vi "WPI_EncoderGet.vi"(8 "error in (no error)":errorcluster, 11 "EncoderDevRef":T1={"DevStatus"={"status"=FALSE, "code"=0, "source"=""}, "EncoderIndex"=enum."Invalid", "CounterIndex"=enum."Ctr 1", "DistancePerCount"=2.0, "Decoding Type"=enum."4x"}) -> (0 "error out":errorcluster, 1 "Direction":bool, 2 "Distance":dbl, 3 "EncoderDevRef":T1={"DevStatus"={"status"=FALSE, "code"=0, "source"=""}, "EncoderIndex"=enum."Invalid", "CounterIndex"=enum."Ctr 1", "DistancePerCount"=2.0, "Decoding Type"=enum."4x"}, 4 "Rate":dbl, 6 "Stopped":bool)   [LabVIEW 2017]
doc: "Returns information about the count, direction, and period of the encoder you specify, as well as whether the encoder is stopped.\n\nThis software is licensed. Open the labview\\readme\\WPI Robotics Library Open Source License.txt file for more information."
uses:
  <vilib>/Rock Robotics/WPI/Encoder/WPI_EncoderDevRef.ctl
  <vilib>/Rock Robotics/SystemInterfaces/Encoder/FPGA_EncoderIdx.ctl
  <vilib>/Rock Robotics/SystemInterfaces/Counter/FPGA_CounterCtrSystemIndex.ctl
  <vilib>/Rock Robotics/WPI/Encoder/WPI_EncoderType.ctl
  <instrlib>/Maxon Encoder/HAIOL/Maxon Encoder.lvclass
  <vilib>/Rock Robotics/SystemInterfaces/Encoder/FPGA_EncoderOpen WO Configuration.vi
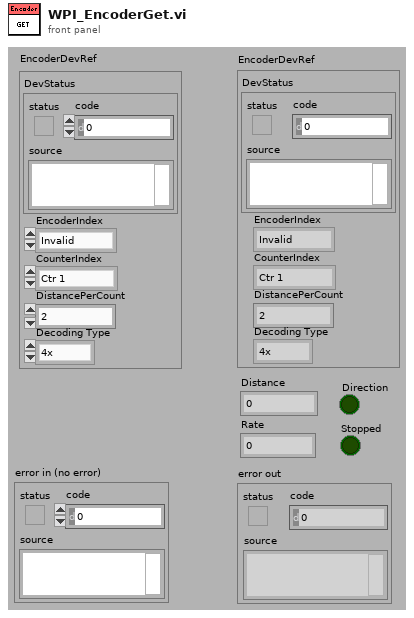
[diagram p1: front panel]
types:
  T1 = typedef "WPI_EncoderDevRef.ctl" = cluster{"DevStatus":errorcluster, "EncoderIndex":T2, "CounterIndex":T3, "DistancePerCount":dbl, "Decoding Type":T4}
  T2 = typedef "FPGA_EncoderIdx.ctl" = enum8{"Enc 0", "Enc 1", "Enc 2", "Enc 3", "Enc 4", "Enc 5", "Enc 6", "Enc 7", "Invalid"}
  T3 = typedef "FPGA_CounterCtrSystemIndex.ctl" = enum8{"Ctr 0", "Ctr 1", "Ctr 2", "Ctr 3", "Ctr 4", "Ctr 5", "Ctr 6", "Ctr 7", "Invalid"}
  T4 = typedef "WPI_EncoderType.ctl" = enum16{"1x", "2x", "4x"}
  T5 = typedef "FPGA_CounterCtrDevRef.ctl" = cluster{"DevStatus":errorcluster, "CntIndex":T3}
  T6 = typedef "FPGA_EncoderDevRef.ctl" = cluster{"EncoderIndex":T2, "DevStatus":errorcluster}
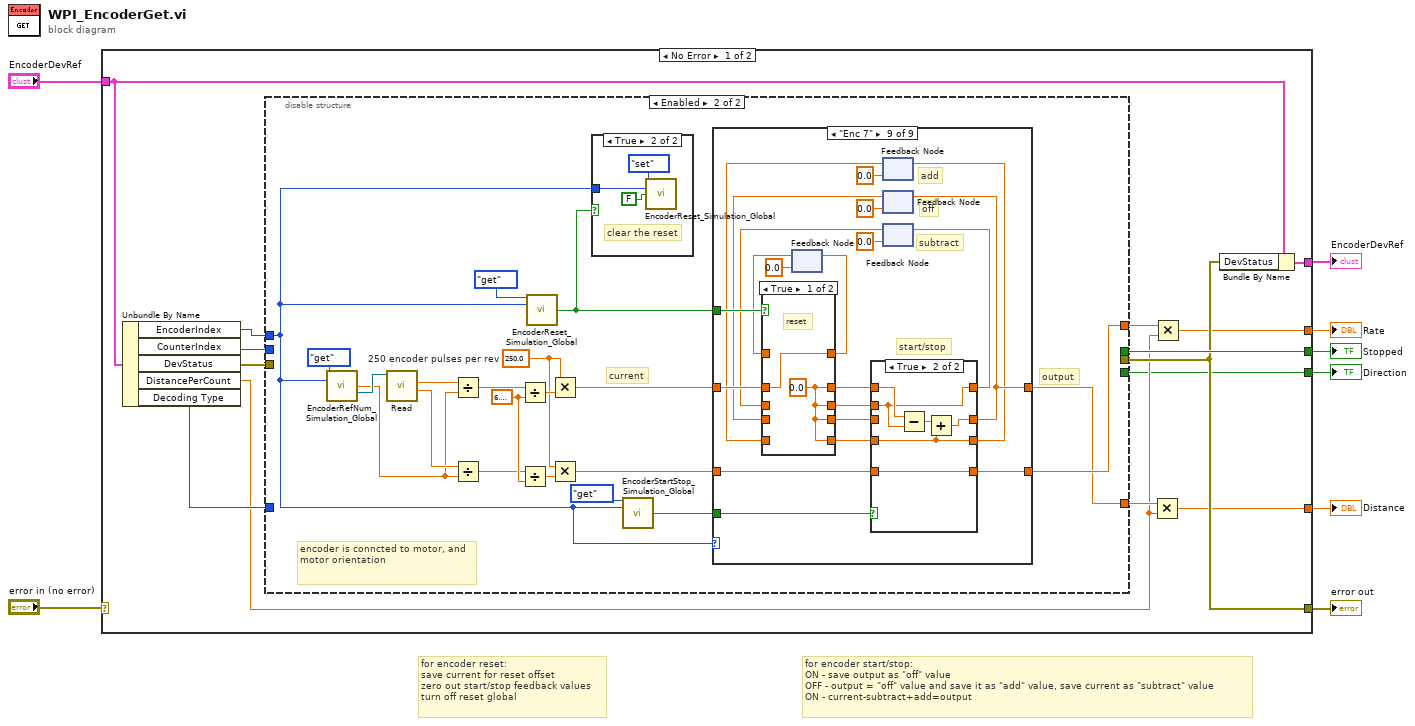
[diagram p0: block diagram]
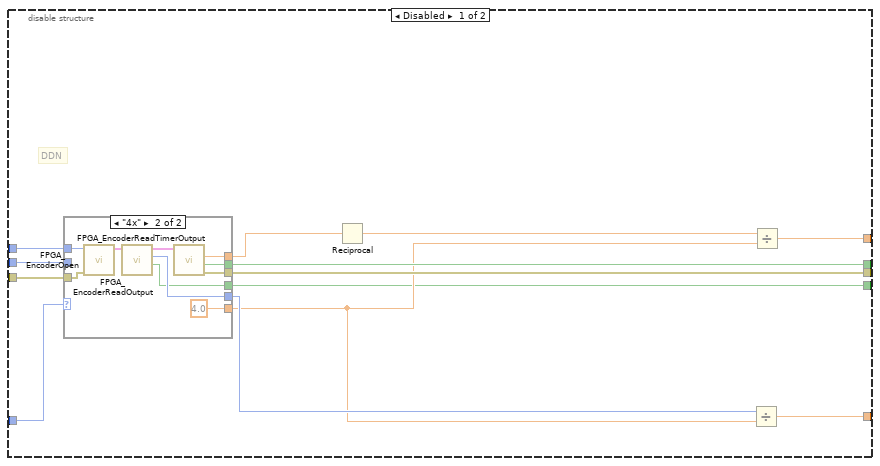
[diagram p2: hidden frame]
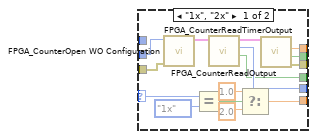
[diagram p3: hidden frame]
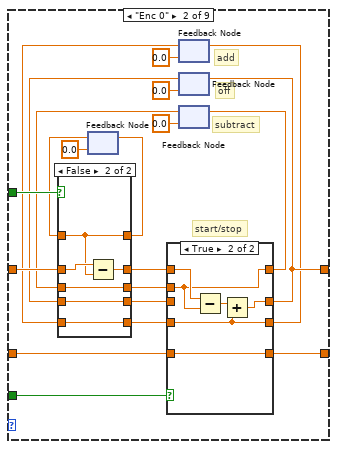
[diagram p6: hidden frame]
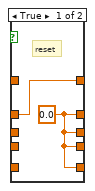
[diagram p7: hidden frame]
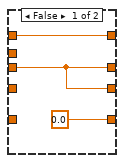
[diagram p8: hidden frame]
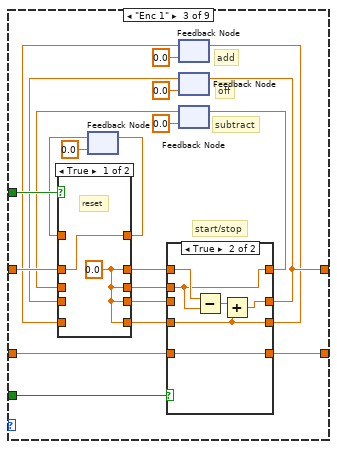
[diagram p9: hidden frame]
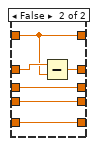
[diagram p10: hidden frame]
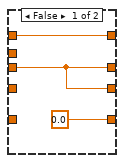
[diagram p11: hidden frame]
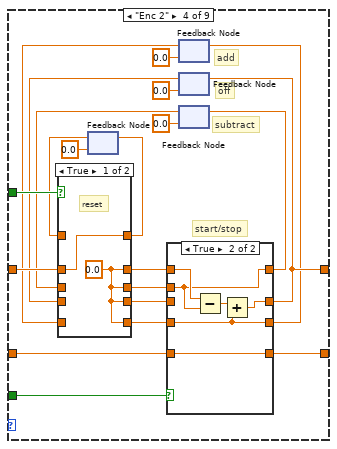
[diagram p12: hidden frame]
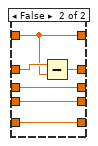
[diagram p13: hidden frame]
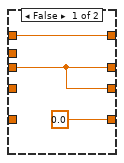
[diagram p14: hidden frame]
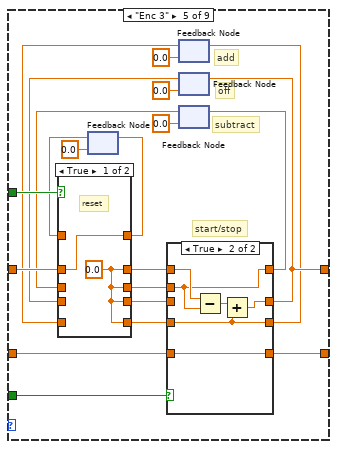
[diagram p15: hidden frame]
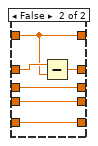
[diagram p16: hidden frame]
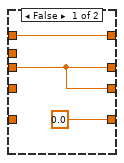
[diagram p17: hidden frame]
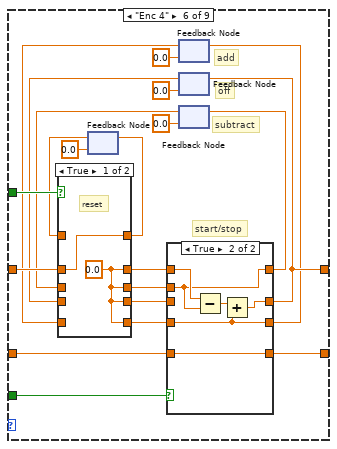
[diagram p18: hidden frame]
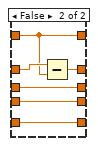
[diagram p19: hidden frame]
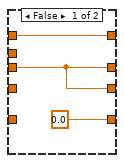
[diagram p20: hidden frame]
diagram:
  # "for encoder reset:\nsave current for reset offset\nzero out start/stop feedback values\nturn off reset global"
  # "for encoder start/stop:\nON - save output as \"off\" value\nOFF - output = \"off\" value and save it as \"add\" value, save current as \"subtract\" value\nON - current-subtract+add=output"
  n1 = case shown="No Error" "error in (no error)" {
    selector: "error in (no error)" -> [_ w390]
    tunnel: "EncoderDevRef" -> [w19 w392]
    tunnel: [w10 _] -> w4
    tunnel: [w15 w390] -> w6
    tunnel: [w22 w391] -> w5
    tunnel: [w12 _] -> w3
    tunnel: [w21 _] -> w2
    tunnel: [w11 _] -> w1
    frame No Error {
      n2 = Unbundle By Name(w19) -> ("EncoderIndex"=w9:T2, "CounterIndex"=w17:T3, "DevStatus"=w18:errorcluster, "DistancePerCount"=w13:dbl, "Decoding Type"=w16:T4)
      n3 = disable-structure shown="Enabled" {
        disable-tunnel: w9 -> [w35 w63]
        disable-tunnel: [w34 _] -> w21
        disable-tunnel: [w33 w62] -> w20
        disable-tunnel: w18 -> [w31 _]
        disable-tunnel: w17 -> [w30 _]
        disable-tunnel: w16 -> [w29 _]
        disable-tunnel: [w28 _] -> w15
        disable-tunnel: [w27 w65] -> w14
        disable-tunnel: [w23 _] -> w12
        frame Disabled {
          # "DDN"
          n4 = case shown="\"4x\"" w29 {
            selector: w29 -> [w49 _]
            tunnel: w35 -> [_ w60]
            tunnel: [w42 w58] -> w32
            tunnel: [w38 w56] -> w34
            tunnel: [w39 w55] -> w24
            tunnel: [w41 w54] -> w23
            tunnel: [w40 w53] -> w28
            tunnel: [w50 4.0] -> w25
            tunnel: w31 -> [w36 w51]
            tunnel: w30 -> [w37 _]
            frame "1x", "2x" {
              n5 = call <vilib>:"FPGA_CounterOpen WO Configuration.vi"("error in"=w36, "CntIndex"=w37) -> ("Ctr Ref"=w43:T5)  [unwired: 1 in, 8 out]
              n6 = Equal?(x=w49, y=WPI_EncoderType."1x") -> (x = y?=w45:bool)
              n7 = call <vilib>:"FPGA_CounterReadOutput.vi"("Ctr Ref in"=w43) -> ("Direction"=w41:bool, "Value"=w42:i32, "Ctr Ref out"=w44:T5)  [unwired: 1 in, 7 out]
              n8 = Select(t=1.0, s=w45, f=2.0) -> (s? t:f=w50:dbl)
              n9 = call <vilib>:"FPGA_CounterReadTimerOutput.vi"("Ctr Ref in"=w44) -> ("error out"=w40:errorcluster, "Stalled"=w38:bool, "Period (s)"=w39:dbl)  [unwired: 1 in, 7 out]
            }
            frame "4x" {
              n10 = call-poly <vilib>:"FPGA_EncoderOpen.vi"("DeviceStatus"=w51, "EncoderIndex"=w60) -> ("Encoder Reference"=w59:T6)  [unwired: 1 in, 8 out]
              n11 = call <vilib>:"FPGA_EncoderReadOutput.vi"("EncoderDevRef"=w59) -> ("Direction"=w54:bool, "Value"=w58:i32, "EncoderDevRef"=w57:T6)  [unwired: 1 in, 7 out]
              n12 = call <vilib>:"FPGA_EncoderReadTimerOutput.vi"("EncoderDevRef"=w57) -> ("error out"=w53:errorcluster, "Stalled"=w56:bool, "Period (s)"=w55:dbl)  [unwired: 1 in, 7 out]
            }
          }
          n13 = Reciprocal(x=w24) -> (1/x=w26:dbl)
          n14 = Divide(x=w32, y=w25) -> (x/y=w33:dbl)
          n15 = Divide(x=w26, y=w25) -> (x/y=w27:dbl)
        }
        frame Enabled {
          w75 = 250.0  # 250 encoder pulses per rev
          w76 = 6.283185307179586
          # "output"
          # "current"
          # "encoder is conncted to motor, and motor orientation"
          n16 = call <vilib>:"EncoderRefNum_Simulation_Global.vi"("menu"=enum16{"set", "get", "delete"}."get", "Encoder"=w63) -> ("Rate out"=w70:dbl, "Maxon Encoder Get"=w79:refnum<class "Maxon Encoder.lvclass">)  [unwired: 11 in, 1 out]
          n17 = call-dynamic "Read.vi"("Maxon Encoder in"=w79) -> ("Velocity (rad/Sec)"=w72:dbl, "Angular Position (rad)"=w74:dbl)  [unwired: 7 in, 2 out]
          n18 = Divide(x=w74, y=w70) -> (x/y=w73:dbl)
          n19 = Divide(x=w72, y=w70) -> (x/y=w71:dbl)
          n20 = Divide(x=w73, y=w76) -> (x/y=w78:dbl)
          n21 = Divide(x=w71, y=w76) -> (x/y=w77:dbl)
          n22 = call <vilib>:"EncoderReset_Simulation_Global.vi"("menu"=enum16{"set", "get", "delete"}."get", "Encoder Index"=w63) -> ("reset out"=w61:bool)  [unwired: 12 in, 1 out]
          n23 = Multiply(x=w75, y=w78) -> (x*y=w67:dbl)
          n24 = Multiply(x=w75, y=w77) -> (x*y=w66:dbl)
          n25 = case shown="True" w61 {
            tunnel: w63 -> [_ w83]
            frame False {
            }
            frame True {
              # "clear the reset"
              n26 = call <vilib>:"EncoderReset_Simulation_Global.vi"("menu"=enum16{"set", "get", "delete"}."set", "Encoder Index"=w83, "reset in"=FALSE) -> ()  [unwired: 11 in, 2 out]
            }
          }
          n27 = call <vilib>:"EncoderStartStop_Simulation_Global.vi"("menu"=enum16{"set", "get", "delete"}."get", "Encoder Index"=w63) -> ("start/stop out"=w68:bool)  [unwired: 12 in, 1 out]
          n28 = case shown="\"Enc 7\"" w63 {
            tunnel: w68 -> [_ w106 w144 w182 w220 w258 w296 w334 w372]
            tunnel: w67 -> [w85 w95 w133 w171 w209 w247 w285 w323 w361]
            tunnel: w66 -> [w84 w105 w143 w181 w219 w257 w295 w333 w371]
            tunnel: [w85 w99 w137 w175 w213 w251 w289 w327 w365] -> w62
            tunnel: [w84 w104 w142 w180 w218 w256 w294 w332 w370] -> w65
            tunnel: w61 -> [_ w97 w135 w173 w211 w249 w287 w325 w363]
            frame "Invalid" {
            }
            frame "Enc 0" {
              # "start/stop"
              # "add"
              # "subtract"
              # "off"
              n29 = feedback #1(0.0) -> (w93:dbl)
              n30 = feedback #2(0.0) -> (w91:dbl)
              n31 = feedback #3(0.0) -> (w89:dbl)
              n32 = feedback #4(0.0) -> (w86:dbl)
              n33 = case shown="False" w97 {
                tunnel: w95 -> [w108 w114]
                tunnel: [w107 w113] -> w94
                tunnel: w93 -> [_ w112]
                tunnel: [w108 w112] -> w92
                tunnel: w91 -> [_ w111]
                tunnel: [w107 w111] -> w90
                tunnel: [w107 w110] -> w88
                tunnel: w89 -> [_ w110]
                tunnel: [w107 w109] -> w87
                tunnel: w86 -> [_ w109]
                frame True {
                  w107 = 0.0
                  # "reset"
                }
                frame False {
                  n34 = Subtract(x=w114, y=w112) -> (x-y=w113:dbl)
                }
              }
              n35 = feedback-in #1(w92) -> ()
              n36 = case shown="True" w106 {
                tunnel: w94 -> [w116 w122]
                tunnel: [w115 w118] -> w99
                tunnel: w105 -> [_ w123]
                tunnel: [0.0 w123] -> w104
                tunnel: w88 -> [w115 _]
                tunnel: [w116 w121] -> w101
                tunnel: w87 -> [_ w121]
                tunnel: [w115 w119] -> w98
                tunnel: w90 -> [_ w119]
                frame False {
                }
                frame True {
                  n37 = Subtract(x=w122, y=w121) -> (x-y=w120:dbl)
                  n38 = Add(x=w120, y=w119) -> (x+y=w118:dbl)
                }
              }
              n39 = feedback-in #2(w98) -> ()
              n40 = feedback-in #3(w99) -> ()
              n41 = feedback-in #4(w101) -> ()
            }
            frame "Enc 1" {
              # "start/stop"
              # "add"
              # "subtract"
              # "off"
              n42 = feedback #5(0.0) -> (w131:dbl)
              n43 = feedback #6(0.0) -> (w129:dbl)
              n44 = feedback #7(0.0) -> (w127:dbl)
              n45 = feedback #8(0.0) -> (w124:dbl)
              n46 = case shown="True" w135 {
                tunnel: w133 -> [w146 w152]
                tunnel: [w145 w151] -> w132
                tunnel: w131 -> [_ w150]
                tunnel: [w146 w150] -> w130
                tunnel: w129 -> [_ w149]
                tunnel: [w145 w149] -> w128
                tunnel: [w145 w148] -> w126
                tunnel: w127 -> [_ w148]
                tunnel: [w145 w147] -> w125
                tunnel: w124 -> [_ w147]
                frame True {
                  w145 = 0.0
                  # "reset"
                }
                frame False {
                  n47 = Subtract(x=w152, y=w150) -> (x-y=w151:dbl)
                }
              }
              n48 = feedback-in #5(w130) -> ()
              n49 = case shown="True" w144 {
                tunnel: w132 -> [w154 w160]
                tunnel: [w153 w156] -> w137
                tunnel: w143 -> [_ w161]
                tunnel: [0.0 w161] -> w142
                tunnel: w126 -> [w153 _]
                tunnel: [w154 w159] -> w139
                tunnel: w125 -> [_ w159]
                tunnel: [w153 w157] -> w136
                tunnel: w128 -> [_ w157]
                frame False {
                }
                frame True {
                  n50 = Subtract(x=w160, y=w159) -> (x-y=w158:dbl)
                  n51 = Add(x=w158, y=w157) -> (x+y=w156:dbl)
                }
              }
              n52 = feedback-in #6(w136) -> ()
              n53 = feedback-in #7(w137) -> ()
              n54 = feedback-in #8(w139) -> ()
            }
            frame "Enc 2" {
              # "start/stop"
              # "add"
              # "subtract"
              # "off"
              n55 = feedback #9(0.0) -> (w169:dbl)
              n56 = feedback #10(0.0) -> (w167:dbl)
              n57 = feedback #11(0.0) -> (w165:dbl)
              n58 = feedback #12(0.0) -> (w162:dbl)
              n59 = case shown="True" w173 {
                tunnel: w171 -> [w184 w190]
                tunnel: [w183 w189] -> w170
                tunnel: w169 -> [_ w188]
                tunnel: [w184 w188] -> w168
                tunnel: w167 -> [_ w187]
                tunnel: [w183 w187] -> w166
                tunnel: [w183 w186] -> w164
                tunnel: w165 -> [_ w186]
                tunnel: [w183 w185] -> w163
                tunnel: w162 -> [_ w185]
                frame True {
                  w183 = 0.0
                  # "reset"
                }
                frame False {
                  n60 = Subtract(x=w190, y=w188) -> (x-y=w189:dbl)
                }
              }
              n61 = feedback-in #9(w168) -> ()
              n62 = case shown="True" w182 {
                tunnel: w170 -> [w192 w198]
                tunnel: [w191 w194] -> w175
                tunnel: w181 -> [_ w199]
                tunnel: [0.0 w199] -> w180
                tunnel: w164 -> [w191 _]
                tunnel: [w192 w197] -> w177
                tunnel: w163 -> [_ w197]
                tunnel: [w191 w195] -> w174
                tunnel: w166 -> [_ w195]
                frame False {
                }
                frame True {
                  n63 = Subtract(x=w198, y=w197) -> (x-y=w196:dbl)
                  n64 = Add(x=w196, y=w195) -> (x+y=w194:dbl)
                }
              }
              n65 = feedback-in #10(w174) -> ()
              n66 = feedback-in #11(w175) -> ()
              n67 = feedback-in #12(w177) -> ()
            }
            frame "Enc 3" {
              # "start/stop"
              # "add"
              # "subtract"
              # "off"
              n68 = feedback #13(0.0) -> (w207:dbl)
              n69 = feedback #14(0.0) -> (w205:dbl)
              n70 = feedback #15(0.0) -> (w203:dbl)
              n71 = feedback #16(0.0) -> (w200:dbl)
              n72 = case shown="True" w211 {
                tunnel: w209 -> [w222 w228]
                tunnel: [w221 w227] -> w208
                tunnel: w207 -> [_ w226]
                tunnel: [w222 w226] -> w206
                tunnel: w205 -> [_ w225]
                tunnel: [w221 w225] -> w204
                tunnel: [w221 w224] -> w202
                tunnel: w203 -> [_ w224]
                tunnel: [w221 w223] -> w201
                tunnel: w200 -> [_ w223]
                frame True {
                  w221 = 0.0
                  # "reset"
                }
                frame False {
                  n73 = Subtract(x=w228, y=w226) -> (x-y=w227:dbl)
                }
              }
              n74 = feedback-in #13(w206) -> ()
              n75 = case shown="True" w220 {
                tunnel: w208 -> [w230 w236]
                tunnel: [w229 w232] -> w213
                tunnel: w219 -> [_ w237]
                tunnel: [0.0 w237] -> w218
                tunnel: w202 -> [w229 _]
                tunnel: [w230 w235] -> w215
                tunnel: w201 -> [_ w235]
                tunnel: [w229 w233] -> w212
                tunnel: w204 -> [_ w233]
                frame False {
                }
                frame True {
                  n76 = Subtract(x=w236, y=w235) -> (x-y=w234:dbl)
                  n77 = Add(x=w234, y=w233) -> (x+y=w232:dbl)
                }
              }
              n78 = feedback-in #14(w212) -> ()
              n79 = feedback-in #15(w213) -> ()
              n80 = feedback-in #16(w215) -> ()
            }
            frame "Enc 4" {
              # "start/stop"
              # "add"
              # "subtract"
              # "off"
              n81 = feedback #17(0.0) -> (w245:dbl)
              n82 = feedback #18(0.0) -> (w243:dbl)
              n83 = feedback #19(0.0) -> (w241:dbl)
              n84 = feedback #20(0.0) -> (w238:dbl)
              n85 = case shown="True" w249 {
                tunnel: w247 -> [w260 w266]
                tunnel: [w259 w265] -> w246
                tunnel: w245 -> [_ w264]
                tunnel: [w260 w264] -> w244
                tunnel: w243 -> [_ w263]
                tunnel: [w259 w263] -> w242
                tunnel: [w259 w262] -> w240
                tunnel: w241 -> [_ w262]
                tunnel: [w259 w261] -> w239
                tunnel: w238 -> [_ w261]
                frame True {
                  w259 = 0.0
                  # "reset"
                }
                frame False {
                  n86 = Subtract(x=w266, y=w264) -> (x-y=w265:dbl)
                }
              }
              n87 = feedback-in #17(w244) -> ()
              n88 = case shown="True" w258 {
                tunnel: w246 -> [w268 w274]
                tunnel: [w267 w270] -> w251
                tunnel: w257 -> [_ w275]
                tunnel: [0.0 w275] -> w256
                tunnel: w240 -> [w267 _]
                tunnel: [w268 w273] -> w253
                tunnel: w239 -> [_ w273]
                tunnel: [w267 w271] -> w250
                tunnel: w242 -> [_ w271]
                frame False {
                }
                frame True {
                  n89 = Subtract(x=w274, y=w273) -> (x-y=w272:dbl)
                  n90 = Add(x=w272, y=w271) -> (x+y=w270:dbl)
                }
              }
              n91 = feedback-in #18(w250) -> ()
              n92 = feedback-in #19(w251) -> ()
              n93 = feedback-in #20(w253) -> ()
            }
            frame "Enc 5" {
              # "start/stop"
              # "add"
              # "subtract"
              # "off"
              n94 = feedback #21(0.0) -> (w283:dbl)
              n95 = feedback #22(0.0) -> (w281:dbl)
              n96 = feedback #23(0.0) -> (w279:dbl)
              n97 = feedback #24(0.0) -> (w276:dbl)
              n98 = case shown="True" w287 {
                tunnel: w285 -> [w298 w304]
                tunnel: [w297 w303] -> w284
                tunnel: w283 -> [_ w302]
                tunnel: [w298 w302] -> w282
                tunnel: w281 -> [_ w301]
                tunnel: [w297 w301] -> w280
                tunnel: [w297 w300] -> w278
                tunnel: w279 -> [_ w300]
                tunnel: [w297 w299] -> w277
                tunnel: w276 -> [_ w299]
                frame True {
                  w297 = 0.0
                  # "reset"
                }
                frame False {
                  n99 = Subtract(x=w304, y=w302) -> (x-y=w303:dbl)
                }
              }
              n100 = feedback-in #21(w282) -> ()
              n101 = case shown="True" w296 {
                tunnel: w284 -> [w306 w312]
                tunnel: [w305 w308] -> w289
                tunnel: w295 -> [_ w313]
                tunnel: [0.0 w313] -> w294
                tunnel: w278 -> [w305 _]
                tunnel: [w306 w311] -> w291
                tunnel: w277 -> [_ w311]
                tunnel: [w305 w309] -> w288
                tunnel: w280 -> [_ w309]
                frame False {
                }
                frame True {
                  n102 = Subtract(x=w312, y=w311) -> (x-y=w310:dbl)
                  n103 = Add(x=w310, y=w309) -> (x+y=w308:dbl)
                }
              }
              n104 = feedback-in #22(w288) -> ()
              n105 = feedback-in #23(w289) -> ()
              n106 = feedback-in #24(w291) -> ()
            }
            frame "Enc 6" {
              # "start/stop"
              # "add"
              # "subtract"
              # "off"
              n107 = feedback #25(0.0) -> (w321:dbl)
              n108 = feedback #26(0.0) -> (w319:dbl)
              n109 = feedback #27(0.0) -> (w317:dbl)
              n110 = feedback #28(0.0) -> (w314:dbl)
              n111 = case shown="True" w325 {
                tunnel: w323 -> [w336 w342]
                tunnel: [w335 w341] -> w322
                tunnel: w321 -> [_ w340]
                tunnel: [w336 w340] -> w320
                tunnel: w319 -> [_ w339]
                tunnel: [w335 w339] -> w318
                tunnel: [w335 w338] -> w316
                tunnel: w317 -> [_ w338]
                tunnel: [w335 w337] -> w315
                tunnel: w314 -> [_ w337]
                frame True {
                  w335 = 0.0
                  # "reset"
                }
                frame False {
                  n112 = Subtract(x=w342, y=w340) -> (x-y=w341:dbl)
                }
              }
              n113 = feedback-in #25(w320) -> ()
              n114 = case shown="True" w334 {
                tunnel: w322 -> [w344 w350]
                tunnel: [w343 w346] -> w327
                tunnel: w333 -> [_ w351]
                tunnel: [0.0 w351] -> w332
                tunnel: w316 -> [w343 _]
                tunnel: [w344 w349] -> w329
                tunnel: w315 -> [_ w349]
                tunnel: [w343 w347] -> w326
                tunnel: w318 -> [_ w347]
                frame False {
                }
                frame True {
                  n115 = Subtract(x=w350, y=w349) -> (x-y=w348:dbl)
                  n116 = Add(x=w348, y=w347) -> (x+y=w346:dbl)
                }
              }
              n117 = feedback-in #26(w326) -> ()
              n118 = feedback-in #27(w327) -> ()
              n119 = feedback-in #28(w329) -> ()
            }
            frame "Enc 7" {
              # "start/stop"
              # "add"
              # "subtract"
              # "off"
              n120 = feedback #29(0.0) -> (w359:dbl)
              n121 = feedback #30(0.0) -> (w357:dbl)
              n122 = feedback #31(0.0) -> (w355:dbl)
              n123 = feedback #32(0.0) -> (w352:dbl)
              n124 = case shown="True" w363 {
                tunnel: w361 -> [w374 w380]
                tunnel: [w373 w379] -> w360
                tunnel: w359 -> [_ w378]
                tunnel: [w374 w378] -> w358
                tunnel: w357 -> [_ w377]
                tunnel: [w373 w377] -> w356
                tunnel: [w373 w376] -> w354
                tunnel: w355 -> [_ w376]
                tunnel: [w373 w375] -> w353
                tunnel: w352 -> [_ w375]
                frame True {
                  w373 = 0.0
                  # "reset"
                }
                frame False {
                  n125 = Subtract(x=w380, y=w378) -> (x-y=w379:dbl)
                }
              }
              n126 = feedback-in #29(w358) -> ()
              n127 = case shown="True" w372 {
                tunnel: w360 -> [w382 w388]
                tunnel: [w381 w384] -> w365
                tunnel: w371 -> [_ w389]
                tunnel: [0.0 w389] -> w370
                tunnel: w354 -> [w381 _]
                tunnel: [w382 w387] -> w367
                tunnel: w353 -> [_ w387]
                tunnel: [w381 w385] -> w364
                tunnel: w356 -> [_ w385]
                frame False {
                }
                frame True {
                  n128 = Subtract(x=w388, y=w387) -> (x-y=w386:dbl)
                  n129 = Add(x=w386, y=w385) -> (x+y=w384:dbl)
                }
              }
              n130 = feedback-in #30(w364) -> ()
              n131 = feedback-in #31(w365) -> ()
              n132 = feedback-in #32(w367) -> ()
            }
          }
        }
      }
      n133 = Multiply(x=w20, y=w13) -> (x*y=w10:dbl)
      n134 = Multiply(x=w14, y=w13) -> (x*y=w11:dbl)
      n135 = Bundle By Name(cluster=w19, "DevStatus"=w15) -> (w22:T1)
    }
    frame Error {
      n136 = Bundle By Name(cluster=w392, "DevStatus"=w390) -> (w391:T1)
    }
  }
  "EncoderDevRef" <- w5
  "error out" <- w6
  "Distance" <- w4
  "Direction" <- w3
  "Rate" <- w1
  "Stopped" <- w2
